vi "Stop Core.vi"(10 "final error code":i32, 11 "UPNCalculatorGUI in":refnum<class "UPNCalculatorGUI.lvclass">) -> (3 "UPNCalculatorGUI out":refnum<class "UPNCalculatorGUI.lvclass">)   [LabVIEW 2016, in "UPNCalculatorGUI Actor.lvlib" / "UPNCalculatorGUI.lvclass"]
doc: "In override VIs of Stop Core.vi, an actor should invoke any code needed to stop all the parallel processes that it created during its run. This includes any nested actors that it created and any other asynchronously running VIs, such as a Time-Delayed Message. It may also include all parallel loops in its Actor Core, although it is acceptable to stop those using a local signal on the Actor Core block diagram that is raised after the Call Parent Node finishes. \n\nThe <b>final error code</b> input tells the actor what error was set when this actor quit. Zero means there was no error. You can use this to decide whether this should be treated as a Normal Stop or an Emergency Stop for the purposes of signaling other actors. In general, any non-zero value should be treated as an Emergency Stop, though a given actor is free to choose other policies. Note that the particular error code 1608 indicates that this actor was itself stopped by an Emergency Stop and should pass that along."
uses:
  UPNCalculatorGUI.lvclass
  UPNCalculatorGUI.lvclass/UPNCalculatorGUI.ctl
  <vilib>/ActorFramework/Message Enqueuer/Message Enqueuer.lvclass/Message Enqueuer.ctl
  <vilib>/ActorFramework/Message Enqueuer/Enqueue.vi
  <vilib>/ActorFramework/Stop Msg/Stop Msg.lvclass
  C:/Program Files (x86)/National Instruments/LabVIEW 2016/vi.lib/ActorFramework/Message/Message.lvclass
  <vilib>/ActorFramework/Message Priority Queue/Priority Enqueue.vi
  <vilib>/ActorFramework/Actor/Actor.lvclass
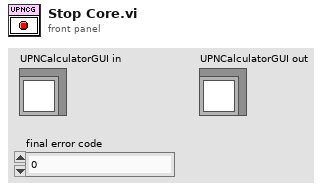
[diagram p1: front panel]
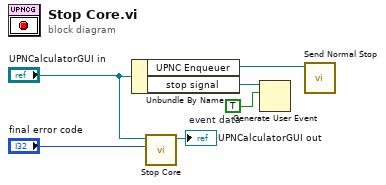
[diagram p0: block diagram]
diagram:
  w2 = TRUE  # event data
  n1 = Unbundle By Name("UPNCalculatorGUI in") -> ("UPNC Enqueuer"=w1:refnum<class "Message Enqueuer.lvclass">, "stop signal"=w3:refnum<user-event>)
  n2 = call-parent "Stop Core.vi"("final error code"="final error code", "Actor in"="UPNCalculatorGUI in") -> ("Actor out"=→"UPNCalculatorGUI out":refnum<class "UPNCalculatorGUI.lvclass">)  [unwired: 9 in]
  n3 = Generate User Event(user event=w3, event data cluster=w2) -> ()  [unwired: 2 in, 2 out]
  n4 = call <vilib>:"Send Normal Stop.vi"("Message Enqueuer"=w1) -> ()  [unwired: 10 in, 1 out]
